vi "MGCC_UnplanISD_main.vi"   [LabVIEW 2016]
doc: "-----------------------------------------------------------------------------------------------------------------------\nCopyright <2019> <The University of Tennessee at Knoxville and the University of Tennessee Research Foundation>\nThis software is released under BSD-3 \nhttps://opensource.org/licenses/BSD-3-Clause \nAdditional license options available at https://utrf.tennessee.edu/industry/sample-agreements/\n-----------------------------------------------------------------------------------------------------------------------"
uses:
  Sub Vis/UnplanISD_Global.vi
  Communication/Global communication.vi
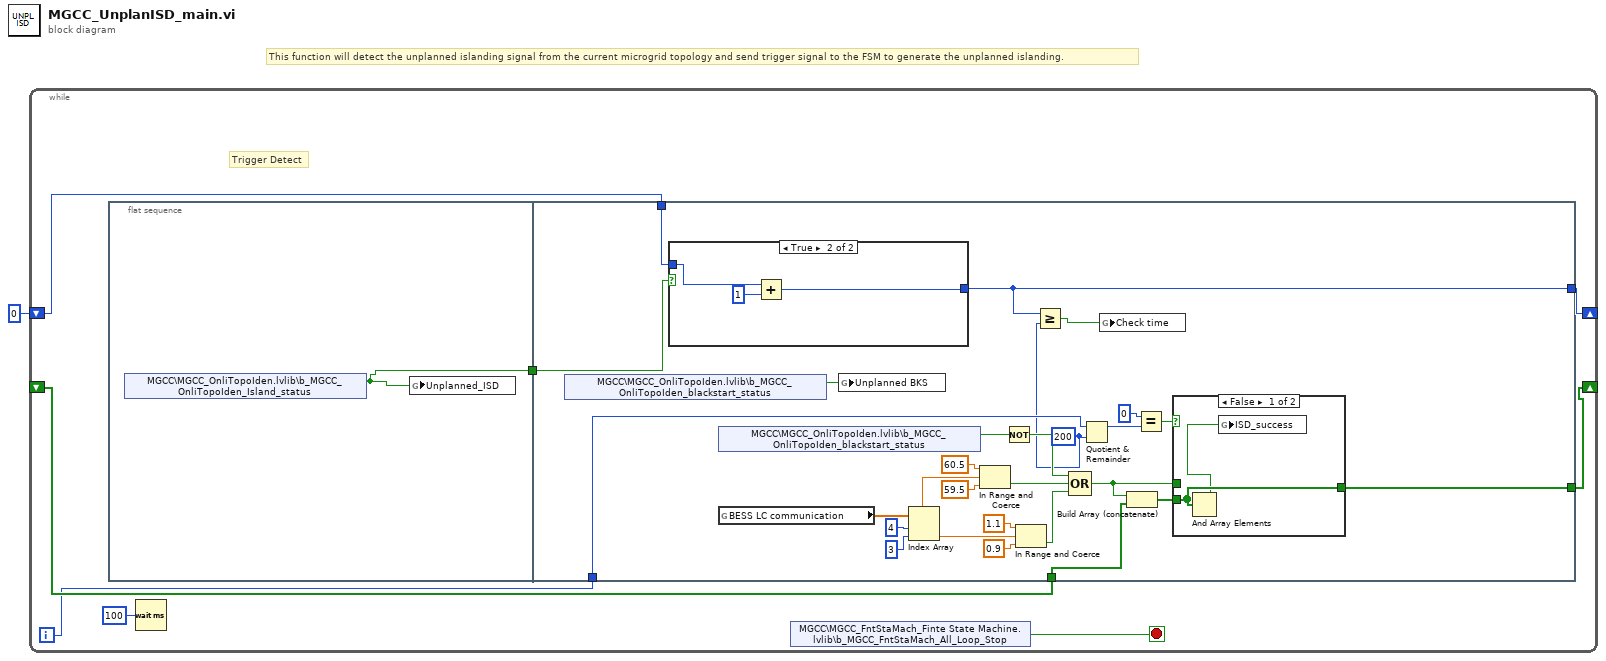
[diagram p0: block diagram]
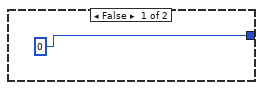
[diagram p2: hidden frame]
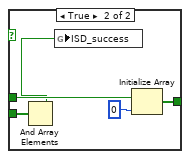
[diagram p3: hidden frame]
diagram:
  # "This function will detect the unplanned islanding signal from the current microgrid topology and send trigger signal to the FSM to generate the unplanned islanding."
  n1 = while {
    shift-right: [w7] -> _
    shift-left: _ -> [w6]
    shift-right: [w3] -> _
    shift-left: 0 -> [w2]
    i -> [w5]
    stop <- w8 stop-if-true
    # "Trigger Detect"
    n2 = flat-sequence {
      tunnel: [w10] -> w4
      tunnel: [w21] -> w7
      tunnel: w6 -> [w28]
      tunnel: w5 -> [w27]
      tunnel: w4 -> [w15]
      tunnel: [w13] -> w3
      tunnel: w2 -> [w14]
      frame #0 {
        n3 = shared-variable "MGCC\\MGCC_OnliTopoIden.lvlib\\b_MGCC_OnliTopoIden_Island_status"() -> (w10:bool)  [unwired: 1 in, 1 out]
        n4 = global write "UnplanISD_Global.vi" "Unplanned_ISD"(w10) -> ()
      }
      frame #1 {
        w12 = 200 ("y")
        n5 = shared-variable "MGCC\\MGCC_OnliTopoIden.lvlib\\b_MGCC_OnliTopoIden_blackstart_status"() -> (w37:bool)  [unwired: 1 in, 1 out]
        n6 = case shown="True" w15 {
          tunnel: [0 w39] -> w13
          tunnel: w14 -> [_ w41]
          frame False {
          }
          frame True {
            n7 = Add(x=w41, y=1) -> (x+y=w39:i32)
          }
        }
        n8 = shared-variable "MGCC\\MGCC_OnliTopoIden.lvlib\\b_MGCC_OnliTopoIden_blackstart_status"() -> (w36:bool)  [unwired: 1 in, 1 out]
        n9 = global read "Global communication.vi" "BESS LC communication"() -> (w20:dbl[])
        n10 = global write "UnplanISD_Global.vi" "Unplanned BKS"(w37) -> ()
        n11 = Index Array(array=w20, index #1=4 ("index"), index #2=3 ("index")) -> (element #1=w18:dbl, element #2=w16:dbl)
        n12 = In Range and Coerce(upper limit=60.5, x=w18, lower limit=59.5) -> (In Range?=w32:bool)  [unwired: 1 out]
        n13 = Not(x=w36) -> (.not. x?=w35:bool)
        n14 = In Range and Coerce(upper limit=1.1, x=w16, lower limit=0.9) -> (In Range?=w29:bool)  [unwired: 1 out]
        n15 = Greater Or Equal?(x=w13, y=w12) -> (x >= y?=w11:bool)
        n16 = Compound Arithmetic op=OR(w35, w32, w29) -> (w22:bool)
        n17 = Quotient & Remainder(x=w27, y=w12) -> (x-y*floor(x/y)=w26:i32)  [unwired: 1 out]
        n18 = global write "UnplanISD_Global.vi" "Check time"(w11) -> ()
        n19 = Build Array (concatenate)(w22, w28) -> (w23:bool[])
        n20 = Equal?(x=0, y=w26) -> (x = y?=w24:bool)
        n21 = case shown="False" w24 {
          tunnel: w23 -> [w43 w48]
          tunnel: w22 -> [_ w46]
          tunnel: [w43 w45] -> w21
          frame False {
            n22 = And Array Elements(Boolean array=w43) -> (logical AND=w42:bool)
            n23 = global write "UnplanISD_Global.vi" "ISD_success"(w42) -> ()
          }
          frame True {
            n24 = And Array Elements(Boolean array=w48) -> (logical AND=w44:bool)
            n25 = global write "UnplanISD_Global.vi" "ISD_success"(w44) -> ()
            n26 = Initialize Array(w46, 0 ("dimension size")) -> (w45:bool[])
          }
        }
      }
    }
    n27 = Wait (ms)(milliseconds to wait=u32 100) -> ()  [unwired: 1 out]
    n28 = shared-variable "MGCC\\MGCC_FntStaMach_Finte State Machine.lvlib\\b_MGCC_FntStaMach_All_Loop_Stop"() -> (w8:bool)  [unwired: 1 in, 1 out]
  }
